vi "CAN Frame Cluster to Array.vi"(1 "CAN Frame Cluster In":T1={"Timestamp"=0, "Identifier"=0, "Type"=0, "InfoA"=0, "InfoB"=0, "DataLength"=0, "Data"=[0, 0, 0, 0, 0, 0, 0, 0]} {"Data" format="%.0x"; "DataLength" format="%.0x"; "InfoB" format="%.0x"; "InfoA" format="%.0x"; "Type" format="%.0x"; "Identifier" format="%.0x"; "Timestamp" format="%.0x"}) -> (0 "CAN Frame Array Out":u32[](array[numeric]))   [LabVIEW 2016]
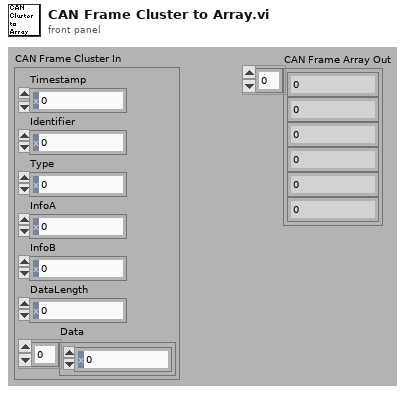
[diagram p1: front panel]
types:
  T1 = cluster{"Timestamp":u64, "Identifier":u32, "Type":u8, "InfoA":u8, "InfoB":u8, "DataLength":u8, "Data":u8[]}
  T2 = cluster{"Data[0]":u8, "Data[1]":u8, "Data[2]":u8, "Data[3]":u8, "Data[4]":u8, "Data[5]":u8, "Data[6]":u8, "Data[7]":u8}
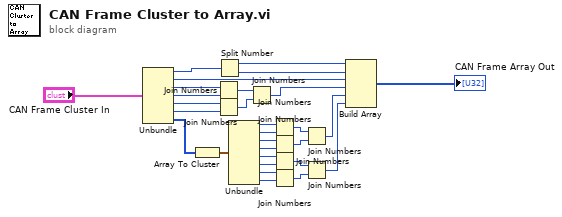
[diagram p0: block diagram]
diagram:
  n1 = Unbundle("CAN Frame Cluster In") -> ("Timestamp"=w5:u64, "Identifier"=w12:u32, "Type"=w6:u8, "InfoA"=w7:u8, "InfoB"=w8:u8, "DataLength"=w9:u8, "Data"=w3:u8[])
  n2 = Array To Cluster(array=w3) -> (cluster=w16:T2)
  n3 = Join Numbers(hi=w7, lo=w6) -> ((hi.lo)=w13:u16)
  n4 = Join Numbers(hi=w8, lo=w9) -> ((hi.lo)=w14:u16)
  n5 = Split Number(x=w5) -> (hi(x)=w10:u32, lo(x)=w11:u32)
  n6 = Unbundle(w16) -> ("Data[0]"=w17:u8, "Data[1]"=w18:u8, "Data[2]"=w19:u8, "Data[3]"=w20:u8, "Data[4]"=w21:u8, "Data[5]"=w22:u8, "Data[6]"=w23:u8, "Data[7]"=w24:u8)
  n7 = Join Numbers(hi=w13, lo=w14) -> ((hi.lo)=w15:u32)
  n8 = Join Numbers(hi=w17, lo=w18) -> ((hi.lo)=w25:u16)
  n9 = Join Numbers(hi=w19, lo=w20) -> ((hi.lo)=w26:u16)
  n10 = Join Numbers(hi=w21, lo=w22) -> ((hi.lo)=w27:u16)
  n11 = Join Numbers(hi=w23, lo=w24) -> ((hi.lo)=w28:u16)
  n12 = Join Numbers(hi=w25, lo=w26) -> ((hi.lo)=w2:u32)
  n13 = Join Numbers(hi=w27, lo=w28) -> ((hi.lo)=w1:u32)
  n14 = Build Array(w10, w11, w12, w15, w2, w1) -> (→"CAN Frame Array Out":u32[])
